vi "Parse SSH_FXP_ATTRS.vi"(8 "error in":errorcluster, 11 "payload":u8[](array[numeric])) -> (0 "error out":errorcluster, 3 "file attributes":T1 {"permissions" format="%04o"})   [LabVIEW 2020, in "NI_SFTP.lvlib"]
uses:
  <vilib>/net/SFTP/NI_SFTP.lvlib
  <vilib>/net/SFTP/API/Support/File Attributes.ctl
  <vilib>/net/SFTP/Low Level Connection/Low Level Connection.lvclass
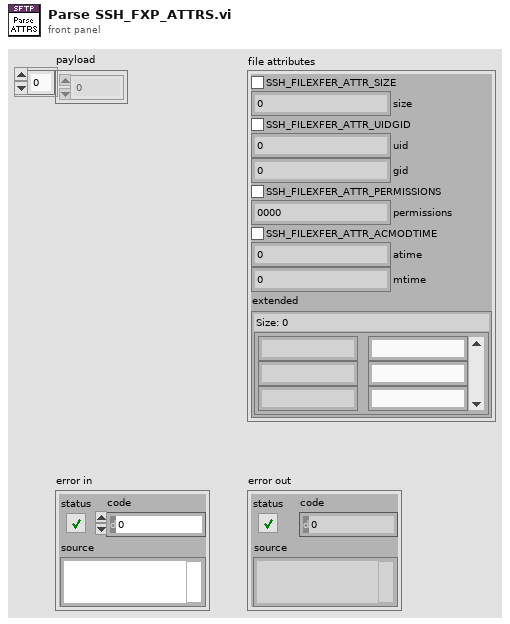
[diagram p1: front panel]
types:
  T1 = typedef "NI_SFTP.lvlib/File Attributes.ctl" = cluster{"SSH_FILEXFER_ATTR_SIZE":bool, "size":u64, "SSH_FILEXFER_ATTR_UIDGID":bool, "uid":u32, "gid":u32, "SSH_FILEXFER_ATTR_PERMISSIONS":bool, "permissions":u32, "SSH_FILEXFER_ATTR_ACMODTIME":bool, "atime":u32, "mtime":u32, "extended":map{string, string}}
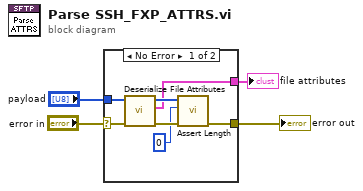
[diagram p0: block diagram]
diagram:
  n1 = case shown="No Error" "error in" {
    selector: "error in" -> [w10 w12]
    tunnel: [w7 w12] -> w3
    tunnel: "payload" -> [w11 _]
    tunnel: [w5 _] -> w1
    frame No Error {
      n2 = call <vilib>:"Deserialize File Attributes.vi"("error in"=w10, "packet"=w11) -> ("error out"=w8:errorcluster, "file attributes"=w5:T1, "packet remaining"=w9:u8[])  [unwired: 7 in]
      n3 = call <vilib>:"Assert Length.vi"("error in"=w8, "asserted length"=u32 0, "string in"=w9) -> ("error out"=w7:errorcluster)  [unwired: 7 in, 1 out]
    }
    frame Error {
    }
  }
  "error out" <- w3
  "file attributes" <- w1
